vi "Engine-User-Host.vi"() -> ()   [LabVIEW 2016]
uses:
  Shared/Typedefs/UserParameter-Array.ctl
  Shared/Typedefs/UserParameter.ctl
  Shared/DSI-Shared.lvlib
panel:
  in  "_Label":string caption="User Plugin (Engine)"
  in  "Enable":bool
  in  "Filename":string caption="User VI File Path (.vi relative to default data directory)"
  out "Error":bool caption="User VI Error"
  in  "Reload":bool
  in  "_User Param":string[][](table) caption="User Parameters"
  in  "_Hidden":enum32{"Page 1"}(tab)
  out "ENG|User|ParamNames":string[](array[string])
  in  "ENG|User|ParamValues":sgl[](array[numeric])
  out "ENG|User|Results":T1=[{"Name"="", "Value"=0.0}, {"Name"="", "Value"=0.0}, {"Name"="", "Value"=0.0}, {"Name"="", "Value"=0.0}, {"Name"="", "Value"=0.0}, {"Name"="", "Value"=0.0}, {"Name"="", "Value"=0.0}, {"Name"="", "Value"=0.0}, {"Name"="", "Value"=0.0}, {"Name"="", "Value"=0.0}, {"Name"="", "Value"=0.0}, {"Name"="", "Value"=0.0}, {"Name"="", "Value"=0.0}, {"Name"="", "Value"=0.0}, {"Name"="", "Value"=0.0}, {"Name"="", "Value"=0.0}, {"Name"="", "Value"=0.0}, {"Name"="", "Value"=0.0}, {"Name"="", "Value"=0.0}, {"Name"="", "Value"=0.0}, {"Name"="", "Value"=0.0}, {"Name"="", "Value"=0.0}, {"Name"="", "Value"=0.0}, {"Name"="", "Value"=0.0}, {"Name"="", "Value"=0.0}, {"Name"="", "Value"=0.0}, {"Name"="", "Value"=0.0}, {"Name"="", "Value"=0.0}, {"Name"="", "Value"=0.0}, {"Name"="", "Value"=0.0}, {"Name"="", "Value"=0.0}, {"Name"="", "Value"=0.0}, {"Name"="", "Value"=0.0}, {"Name"="", "Value"=0.0}, {"Name"="", "Value"=0.0}, {"Name"="", "Value"=0.0}, {"Name"="", "Value"=0.0}, {"Name"="", "Value"=0.0}, {"Name"="", "Value"=0.0}, {"Name"="", "Value"=0.0}, {"Name"="", "Value"=0.0}, {"Name"="", "Value"=0.0}, {"Name"="", "Value"=0.0}, {"Name"="", "Value"=0.0}, {"Name"="", "Value"=0.0}, {"Name"="", "Value"=0.0}, {"Name"="", "Value"=0.0}, {"Name"="", "Value"=0.0}, {"Name"="", "Value"=0.0}, {"Name"="", "Value"=0.0}, {"Name"="", "Value"=0.0}, {"Name"="", "Value"=0.0}, {"Name"="", "Value"=0.0}, {"Name"="", "Value"=0.0}, {"Name"="", "Value"=0.0}, {"Name"="", "Value"=0.0}, {"Name"="", "Value"=0.0}, {"Name"="", "Value"=0.0}, {"Name"="", "Value"=0.0}, {"Name"="", "Value"=0.0}, {"Name"="", "Value"=0.0}, {"Name"="", "Value"=0.0}, {"Name"="", "Value"=0.0}, {"Name"="", "Value"=0.0}, {"Name"="", "Value"=0.0}, {"Name"="", "Value"=0.0}, {"Name"="", "Value"=0.0}, {"Name"="", "Value"=0.0}, {"Name"="", "Value"=0.0}, {"Name"="", "Value"=0.0}, {"Name"="", "Value"=0.0}, {"Name"="", "Value"=0.0}, {"Name"="", "Value"=0.0}, {"Name"="", "Value"=0.0}, {"Name"="", "Value"=0.0}, {"Name"="", "Value"=0.0}, {"Name"="", "Value"=0.0}, {"Name"="", "Value"=0.0}, {"Name"="", "Value"=0.0}, {"Name"="", "Value"=0.0}, {"Name"="", "Value"=0.0}, {"Name"="", "Value"=0.0}, {"Name"="", "Value"=0.0}, {"Name"="", "Value"=0.0}, {"Name"="", "Value"=0.0}, {"Name"="", "Value"=0.0}, {"Name"="", "Value"=0.0}, {"Name"="", "Value"=0.0}, {"Name"="", "Value"=0.0}, {"Name"="", "Value"=0.0}, {"Name"="", "Value"=0.0}, {"Name"="", "Value"=0.0}, {"Name"="", "Value"=0.0}, {"Name"="", "Value"=0.0}, {"Name"="", "Value"=0.0}, {"Name"="", "Value"=0.0}, {"Name"="", "Value"=0.0}, {"Name"="", "Value"=0.0}, {"Name"="", "Value"=0.0}, {"Name"=" ", "Value"=0.0}]
  out "_User Results":string[][](table) caption="User Results"
  # "Enable Plugin"
  # "File Path (.lvclass relative to default data directory)"
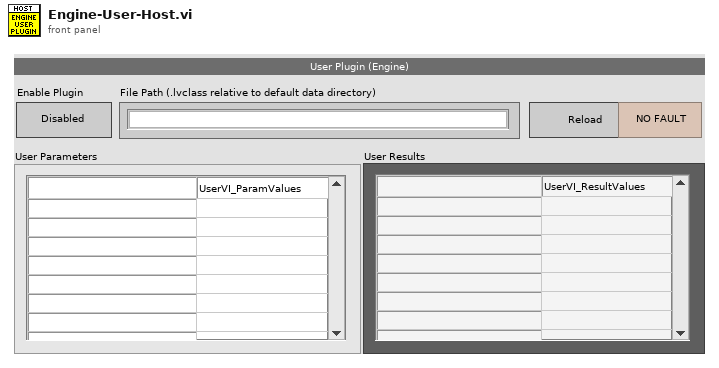
[diagram p1: front panel]
types:
  T1 = typedef "DSI-Shared.lvlib/UserParameter-Array.ctl" = T2[]
  T2 = typedef "DSI-Shared.lvlib/UserParameter.ctl" = cluster{"Name":string, "Value":dbl}
  T3 = typedef "LVRectTypeDef.ctl" = cluster{"Left":i16, "Top":i16, "Right":i16, "Bottom":i16}
  T4 = typedef "LVBoundsTypeDef.ctl" = cluster{"Width":u32, "Height":u32}
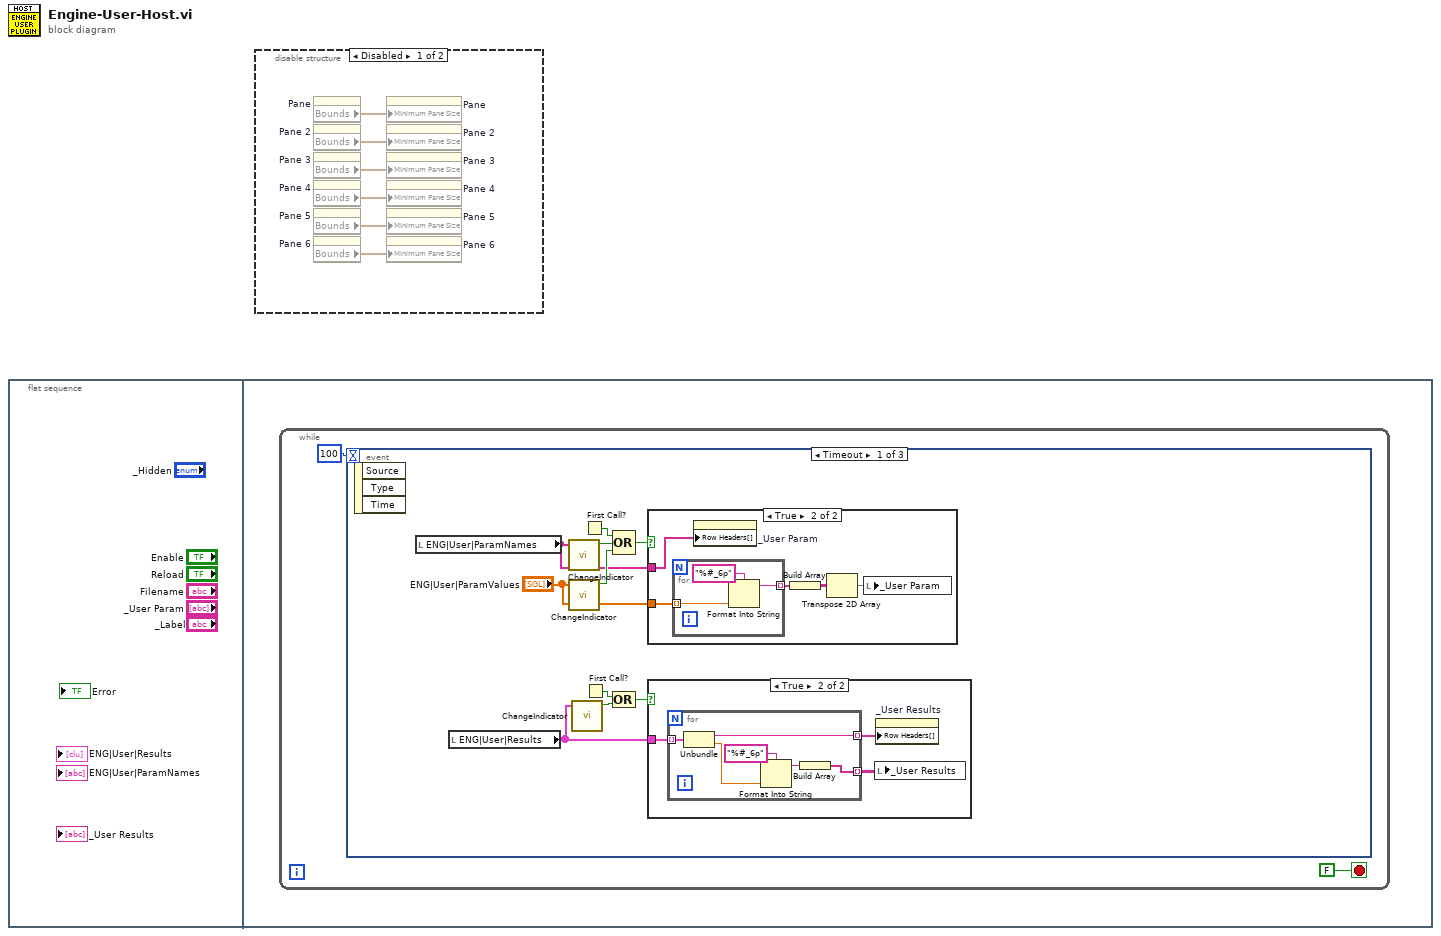
[diagram p0: block diagram]
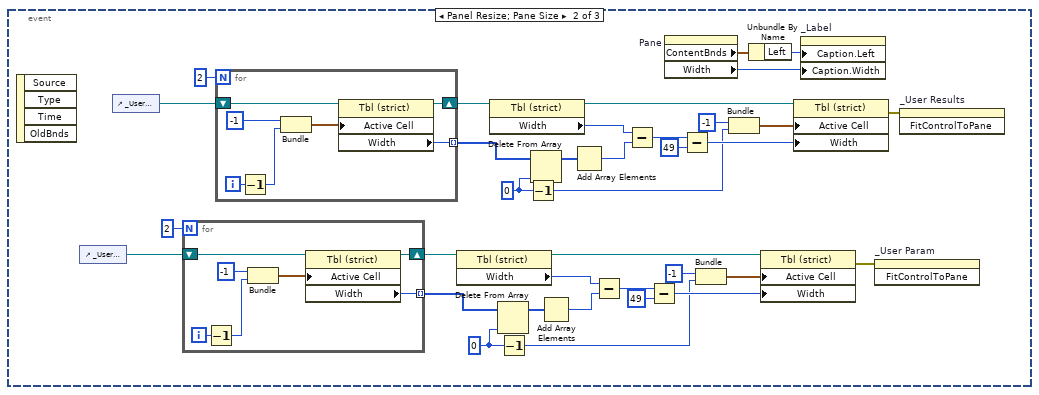
[diagram p5: hidden frame]
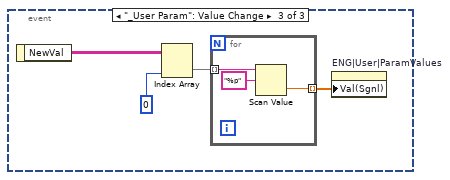
[diagram p6: hidden frame]
diagram:
  n1 = flat-sequence {
    frame #0 {
    }
    frame #1 {
      n2 = while {
        stop <- FALSE stop-if-true
        n3 = event shown="[0] Timeout" {
          selector: _ -> [_ _ _]
          dyn-events: _ -> [_ _ _]
          timeout: 100 ("millisecond multiple") -> [_ _ _]
          event Timeout {
            n4 = event-data() -> ()  [unwired: 1 in, 3 out]
            n5 = local read "ENG|User|ParamNames"() -> (w5:string[])
            n6 = local read "ENG|User|Results"() -> (w4:T1)
            n7 = call "ChangeIndicator.vi"("Input"=w5) -> ("Change"=w10:bool)  [unwired: 9 in]
            n8 = call "ChangeIndicator.vi"("Input"="ENG|User|ParamValues") -> ("Change"=w9:bool)  [unwired: 9 in]
            n9 = call "ChangeIndicator.vi"("Input"=w4) -> ("Change"=w7:bool)  [unwired: 9 in]
            n10 = First Call?() -> (First Call?: T/F=w6:bool)
            n11 = First Call?() -> (First Call?: T/F=w3:bool)
            n12 = Compound Arithmetic op=OR(w6, w10, w9) -> (w8:bool)
            n13 = Compound Arithmetic op=OR(w3, w7) -> (w12:bool)
            n14 = case shown="True" w8 {
              tunnel: "ENG|User|ParamValues" -> [_ w13]
              tunnel: w5 -> [_ w15]
              frame False {
              }
              frame True {
                n15 = for {
                  tunnel: w13 -> [w20] mode=indexing
                  tunnel: [w19] -> w14 mode=indexing
                  n16 = Format Into String(format string="%#_6p", w20) -> (resulting string=w19:string)  [unwired: 2 in, 1 out]
                }
                n17 = property on="_User Param" class="Tbl (strict)"("Row Headers[]"=w15) -> ()  [unwired: 2 in, 2 out]
                n18 = Build Array(w14) -> (w17:string[][])
                n19 = Transpose 2D Array(2D array=w17) -> (transposed array=w16:string[][])
                n20 = local write "_User Param"(w16) -> ()
              }
            }
            n21 = case shown="True" w12 {
              tunnel: w4 -> [_ w23]
              frame False {
              }
              frame True {
                n22 = for {
                  tunnel: [w27] -> w21 mode=indexing
                  tunnel: w23 -> [w29] mode=indexing
                  tunnel: [w28] -> w22 mode=indexing
                  n23 = Unbundle(w29) -> ("Name"=w28:string, "Value"=w24:dbl)
                  n24 = Format Into String(format string="%#_6p", w24) -> (resulting string=w25:string)  [unwired: 2 in, 1 out]
                  n25 = Build Array(w25) -> (w27:string[])
                }
                n26 = local write "_User Results"(w21) -> ()
                n27 = property on="_User Results" class="Tbl (strict)"("Row Headers[]"=w22) -> ()  [unwired: 2 in, 2 out]
              }
            }
          }
          event Panel Resize; Pane Size {
            w41 = 0 ("index")
            w59 = 0 ("index")
            n28 = event-data() -> ()  [unwired: 1 in, 4 out]
            n29 = control-ref of="_User Param"() -> (w63:refnum<vi>)
            n30 = control-ref of="_User Results"() -> (w37:refnum<vi>)
            n31 = for {
              N: 2 -> [_]
              shift-right: [w75] -> w54
              shift-left: w63 -> [w76]
              tunnel: [w73] -> w55 mode=indexing
              i -> [w78]
              n32 = Decrement(x=w78) -> (x-1=w72:i32)
              n33 = Bundle(-1, w72) -> (w74:cluster{i32, i32})  [unwired: 1 in]
              n34 = property class="Tbl (strict)"(reference=w76, "Active Cell"=w74) -> (reference out=w75:refnum<vi>, "Width"=w73:u32)  [unwired: 1 in, 1 out]
            }
            n35 = for {
              N: 2 -> [_]
              shift-right: [w68] -> w46
              shift-left: w37 -> [w69]
              tunnel: [w66] -> w45 mode=indexing
              i -> [w71]
              n36 = Decrement(x=w71) -> (x-1=w65:i32)
              n37 = Bundle(-1, w65) -> (w67:cluster{i32, i32})  [unwired: 1 in]
              n38 = property class="Tbl (strict)"(reference=w69, "Active Cell"=w67) -> (reference out=w68:refnum<vi>, "Width"=w66:u32)  [unwired: 1 in, 1 out]
            }
            n39 = property on="Property Node" class="Tbl (strict)"(reference=w54) -> (reference out=w53:refnum<vi>, "Width"=w52:u32)  [unwired: 1 in, 1 out]
            n40 = property on="Property Node" class="Tbl (strict)"(reference=w46) -> (reference out=w47:refnum<vi>, "Width"=w48:u32)  [unwired: 1 in, 1 out]
            n41 = Delete From Array(array=w55, index=w59) -> (array with subset deleted=w56:u32[])  [unwired: 1 in, 1 out]
            n42 = Decrement(x=w59) -> (x-1=w50:i32)
            n43 = Decrement(x=w41) -> (x-1=w35:i32)
            n44 = Delete From Array(array=w45, index=w41) -> (array with subset deleted=w44:u32[])  [unwired: 1 in, 1 out]
            n45 = Add Array Elements(numeric array=w56) -> (sum=w57:u32)
            n46 = Add Array Elements(numeric array=w44) -> (sum=w43:u32)
            n47 = Subtract(x=w52, y=w57) -> (x-y=w51:u32)
            n48 = Subtract(x=w48, y=w43) -> (x-y=w49:u32)
            n49 = Subtract(x=w51, y=u32 49) -> (x-y=w61:u32)
            n50 = property on="Pane" class="Pane"() -> ("ContentBnds"=w33:T3, "Width"=w34:u32)  [unwired: 2 in, 2 out]
            n51 = Subtract(x=w49, y=u32 49) -> (x-y=w39:u32)
            n52 = Bundle(-1, w50) -> (w60:cluster{i32, i32})  [unwired: 1 in]
            n53 = Bundle(-1, w35) -> (w40:cluster{i32, i32})  [unwired: 1 in]
            n54 = Unbundle By Name(w33) -> ("Left"=w32:i16)
            n55 = property on="Property Node" class="Tbl (strict)"(reference=w53, "Active Cell"=w60, "Width"=w61) -> (error out=w30:errorcluster)  [unwired: 1 in, 1 out]
            n56 = property on="Property Node" class="Tbl (strict)"(reference=w47, "Active Cell"=w40, "Width"=w39) -> (error out=w31:errorcluster)  [unwired: 1 in, 1 out]
            n57 = property on="_Label" class="Str"("Caption.Left"=w32, "Caption.Width"=w34) -> ()  [unwired: 2 in, 2 out]
            n58 = invoke on="_User Param" class="Tbl (strict)" method="FitControlToPane"(error in=w30) -> ()  [unwired: 2 in, 3 out]
            n59 = invoke on="_User Results" class="Tbl (strict)" method="FitControlToPane"(error in=w31) -> ()  [unwired: 2 in, 3 out]
          }
          event "_User Param": Value Change {
            n60 = event-data() -> ("NewVal"=w82:string[][])  [unwired: 1 in]
            n61 = Index Array(array=w82, index (col)=0 ("disabled index (col)")) -> (element=w80:string[])  [unwired: 1 in]
            n62 = for {
              tunnel: [w85] -> w79 mode=indexing
              tunnel: w80 -> [w84] mode=indexing
              n63 = Scan Value(string=w84, format string="%p") -> (value=w85:dbl)  [unwired: 1 in, 1 out]
            }
            n64 = property on="ENG|User|ParamValues" class="Arr (strict)"("Val(Sgnl)"=w79) -> ()  [unwired: 2 in, 2 out]
          }
        }
      }
    }
  }
  n65 = disable-structure shown="Disabled" {
    frame Disabled {
      n66 = property on="Pane" class="Pane"() -> ("Bounds"=w91:T4)  [unwired: 2 in, 2 out]
      n67 = property on="Pane 2" class="Pane"() -> ("Bounds"=w90:T4)  [unwired: 2 in, 2 out]
      n68 = property on="Pane 3" class="Pane"() -> ("Bounds"=w89:T4)  [unwired: 2 in, 2 out]
      n69 = property on="Pane 4" class="Pane"() -> ("Bounds"=w88:T4)  [unwired: 2 in, 2 out]
      n70 = property on="Pane 5" class="Pane"() -> ("Bounds"=w87:T4)  [unwired: 2 in, 2 out]
      n71 = property on="Pane 6" class="Pane"() -> ("Bounds"=w86:T4)  [unwired: 2 in, 2 out]
      n72 = property on="Pane" class="Pane"("Minimum Pane Size"=w91) -> ()  [unwired: 2 in, 2 out]
      n73 = property on="Pane 2" class="Pane"("Minimum Pane Size"=w90) -> ()  [unwired: 2 in, 2 out]
      n74 = property on="Pane 3" class="Pane"("Minimum Pane Size"=w89) -> ()  [unwired: 2 in, 2 out]
      n75 = property on="Pane 4" class="Pane"("Minimum Pane Size"=w88) -> ()  [unwired: 2 in, 2 out]
      n76 = property on="Pane 5" class="Pane"("Minimum Pane Size"=w87) -> ()  [unwired: 2 in, 2 out]
      n77 = property on="Pane 6" class="Pane"("Minimum Pane Size"=w86) -> ()  [unwired: 2 in, 2 out]
    }
    frame Enabled {
    }
  }
